vi "GTcode_v6 - WithEMGSubVI.vi"() -> ()   [LabVIEW 2016]
uses:
  <vilib>/Utility/config.llb/NI_LVConfig.lvlib
  <vilib>/Utility/config.llb/Write Key (U32).vi
  <vilib>/Utility/config.llb/Read Key (U32).vi
  <vilib>/Analysis/NI_AALBase.lvlib
  <vilib>/Utility/config.llb/Write Key (I32).vi
  <vilib>/Utility/config.llb/Write Key (String).vi
  <vilib>/Utility/config.llb/Read Key (I32).vi
  <vilib>/Utility/config.llb/Write Key (Double).vi
panel:
  in  "InitCH4 Path File":path=path "C:/Users/BUCKLEY-ADMIN/Desktop/DCScode_simulISS_MAP/flex05-4chPascal.dll"
  in  "Stop CH8":path=path "C:/Users/BUCKLEY-ADMIN/Desktop/DCScode_simulISS_MAP/flex05oem8chauto100nsPASCAL_win7.dll"
  in  "Stop Ch 4 Path":path=path "C:/Users/BUCKLEY-ADMIN/Desktop/DCScode_simulISS_MAP/flex05-4chPascal.dll"
  in  "FreeCh4 Path":path=path "C:/Users/BUCKLEY-ADMIN/Desktop/DCScode_simulISS_MAP/flex05-4chPascal.dll"
  in  "initCh4 path":path=path "C:/Users/BUCKLEY-ADMIN/Desktop/DCScode_simulISS_MAP/flex05-4chPascal.dll"
  in  "Ch8 Init channel":path=path "C:/Users/BUCKLEY-ADMIN/Desktop/DCScode_simulISS_MAP/flex05oem8chauto100nsPASCAL_win7.dll"
  in  "FreeCH8 Path":path=path "C:/Users/BUCKLEY-ADMIN/Desktop/DCScode_simulISS_MAP/flex05oem8chauto100nsPASCAL_win7.dll"
  in  "StartCH8 Path":path=path "C:/Users/BUCKLEY-ADMIN/Desktop/DCScode_simulISS_MAP/flex05oem8chauto100nsPASCAL_win7.dll"
  in  "StartCH4":path=path "C:/Users/BUCKLEY-ADMIN/Desktop/DCScode_simulISS_MAP/flex05-4chPascal.dll"
  in  "InitCh8 8 Dectectors Path":path=path "C:/Users/BUCKLEY-ADMIN/Desktop/DCScode_simulISS_MAP/flex05oem8chauto100nsPASCAL_win7.dll"
  in  "init CH4 path":path=path "C:/Users/BUCKLEY-ADMIN/Desktop/DCScode_simulISS_MAP/flex05-4chPascal.dll"
  in  "initCH8 Path":path
  in  "Tab Control":T1(tab)=enum."Real Time Fitting Parameters"
  out "Thermometer":dbl(slide) scale=0.0..100.0
  out "mean":dbl format="%0.1e"
  out "COV":dbl format="%0.1f"
  in  "Fixed Time":bool
  in  "Detector Used":T2(ring)=enum."Det 2"
  in  "Real Time Fitting?":bool=TRUE
  out "g2":cluster{"Delay Time":sgl[], sgl[]}[](graph) caption="Normalized Correlation Function"
  out "Tau":cluster{"tmp":dbl, dbl}(graph) caption="Relative Changes of Flow"
  in  "QUIT":bool
  in  "Clear plots":bool
  in  "Baseline":bool
  in  "MARK\nMark":bool
  in  "Stop":bool
  in  "Sequence Scan":bool
  out "Mark #":u32
  out "Trial #":u32
  out "Frame #":u32
  out "Det 8":sgl format="%.3f"
  out "Det 7":sgl format="%.3f"
  out "Det 6":sgl format="%.3f"
  out "Det 5":sgl format="%.3f"
  out "Det 4":sgl format="%.3f"
  out "Det 3":sgl format="%.3f"
  out "Det 2":sgl format="%.3f"
  out "Det 1":sgl format="%.3f"
  out "Computer Time":string="2010-1-12 23:16:10"
  in  "D1":bool
  in  "D2":bool
  in  "D3":bool
  in  "D4":bool
  in  "D5":bool
  in  "D6":bool
  in  "D7":bool
  in  "D8":bool
  out "Tau 2":T3(graph)={1.6593152555505744e-08, 3.9427894777554196e-08, 4.065716407938411e-08, 1.5135790977358522e-08, 2.4870420100428357e-08, 7.094765128107397e-08, 0.0, 4.1348620928852906e-07, 1.5886917674344795e-08, 4.0280526032721455e-08, -1.0, -1.0} caption="Blood Flow Index (cm2/s)"
  in  "Fixed # of Frames":u32=5
  out "Status":string="Quit"
  in  "Optical Switch OPEN":bool
  in  "Delay between frames(ms)":u32=500
  out "Time Left (ms)":sgl format="%.3f"
  in  "Integration Time (ms)":sgl=1000.0 min=1 max=13000 step=1
  in  "File\nName:":string="test0"
  in  "Data Save Directory:":path=path "C:/data"
  in  "ISS Lasers ON":bool
  in  "Test":bool
  in  "Lines":tag="Dev1/port1/line0:1, Dev1/port1/line3:7"
  in  "Delaytime(ms)":u32=200
  in  "Initialize Correlator":bool
  in  "Detector Select":enum32{"4 Detectors", "8 Detectors"}(radio)=enum."8 Detectors"
  in  "Update Time (ms)\nDO NOT CHANGE!":u32=105 min=1 max=999 step=1
  in  "Laser Input Name":refnum<visa-resource-name>="COM7"
  out "Flow in each detector":dbl[](array[numeric])=[-1.0, -1.0, -1.0, -1.0, -1.0, -1.0, -1.0, -1.0, -1.0, -1.0, -1.0, -1.0]
  in  "Visible Averages":bool[](array[boolean])=[FALSE, FALSE, FALSE, FALSE]
  in  "Avg":bool[][](array[boolean])=[[FALSE, FALSE, FALSE, FALSE, FALSE, FALSE, FALSE, FALSE], [FALSE, FALSE, FALSE, FALSE, FALSE, FALSE, FALSE, FALSE], [FALSE, FALSE, FALSE, FALSE, FALSE, FALSE, FALSE, FALSE], [FALSE, FALSE, FALSE, FALSE, FALSE, FALSE, FALSE, FALSE]]
  in  "rho":dbl[](array[numeric])=[2.5, 2.5, 2.5, 2.5, 2.5, 2.5, 2.5, 2.5, -1.0, -1.0, -1.0, -1.0]
  in  "Other Settings":u32[](array[numeric])=[1, 120, 0, 1] caption="Flow in each detector"
  in  "Initial Guess":dbl[](array[numeric])=[1e-08, 0.5, 0.05, 10.0] caption="Flow in each detector"
  in  "TrialDataFileExtension":string
  in  "UI Data Path":path=path "C:/Users/Tinggroup/Desktop/VRMuscleActivationVisualizer/LabviewFiles/Jake DCScode_GT/BiofeedbackEMGPackage/BiofeedbackData.txt"
  out "4CH?":bool
  out "Detector#":u32=1
  out "Source#":u32=1
  # "kHz"
  # "kHz"
  # "Don't Change these Parameters unless you know clearly what you are doing"
  # "ISS Triggers Setup"
  # "Channel Parameters"
  # "Step1"
  # "Line"
  # "0"
  # "1"
  # "3"
  # "4"
  # "5"
  # "6"
  # "7"
  # "*The number of lines in the list must\nmatch the number of elements in\nthe array."
  # "Step2"
  # "Line"
  # "0"
  # "1"
  # "3"
  # "4"
  # "5"
  # "6"
  # "7"
  # "Step3"
  # "Line"
  # "0"
  # "1"
  # "3"
  # "4"
  # "5"
  # "6"
  # "7"
  # "Line    Signal\n\n0           ISS Trigger (0: OFF, 1: ON)\n1           Flow Laser 1 ON/OFF (0:OFF, 1:ON)\n2           ISS Data Acquisition (0: DONE, 1: NO)\n3           ISS Laser ON/OFF (0: ON, 1: OFF)\n4           Trigger for Marks  (0: OFF, 1: ON)\n5           Flow Laser 2 ON/OFF (0:OFF, 1:ON)\n6           Reserved\n7           Reserved"
  # "Wait ISS Data Acuisition DONE Signal"
  # "Step4"
  # "Step5"
  # "Line"
  # "0"
  # "1"
  # "3"
  # "4"
  # "5"
  # "6"
  # "7"
  # "Flow Lasers Setup"
  # "FROM FRONT PANEL"
  # "Line"
  # "0"
  # "1"
  # "3"
  # "4"
  # "5"
  # "6"
  # "7"
  # "Line"
  # "0"
  # "1"
  # "3"
  # "4"
  # "5"
  # "6"
  # "7"
  # "Det 1"
  # "Det 2"
  # "Det 3"
  # "Det 4"
  # "Det 5"
  # "Det 6"
  # "Det 7"
  # "Det 8"
  # "Avg 1"
  # "Avg 2"
  # "Avg 3"
  # "Avg 4"
  # "Db"
  # "Beta"
  # "Mua"
  # "MuS'"
  # "1"
  # "2"
  # "3"
  # "4"
  # "5"
  # "6"
  # "7"
  # "8"
  # "Avg 1"
  # "Starting Pt"
  # "End Pt"
  # "Approximate"
  # "Variables"
  # "Avg 2"
  # "Avg 3"
  # "Avg 4"
  # "Source Detector  Separations"
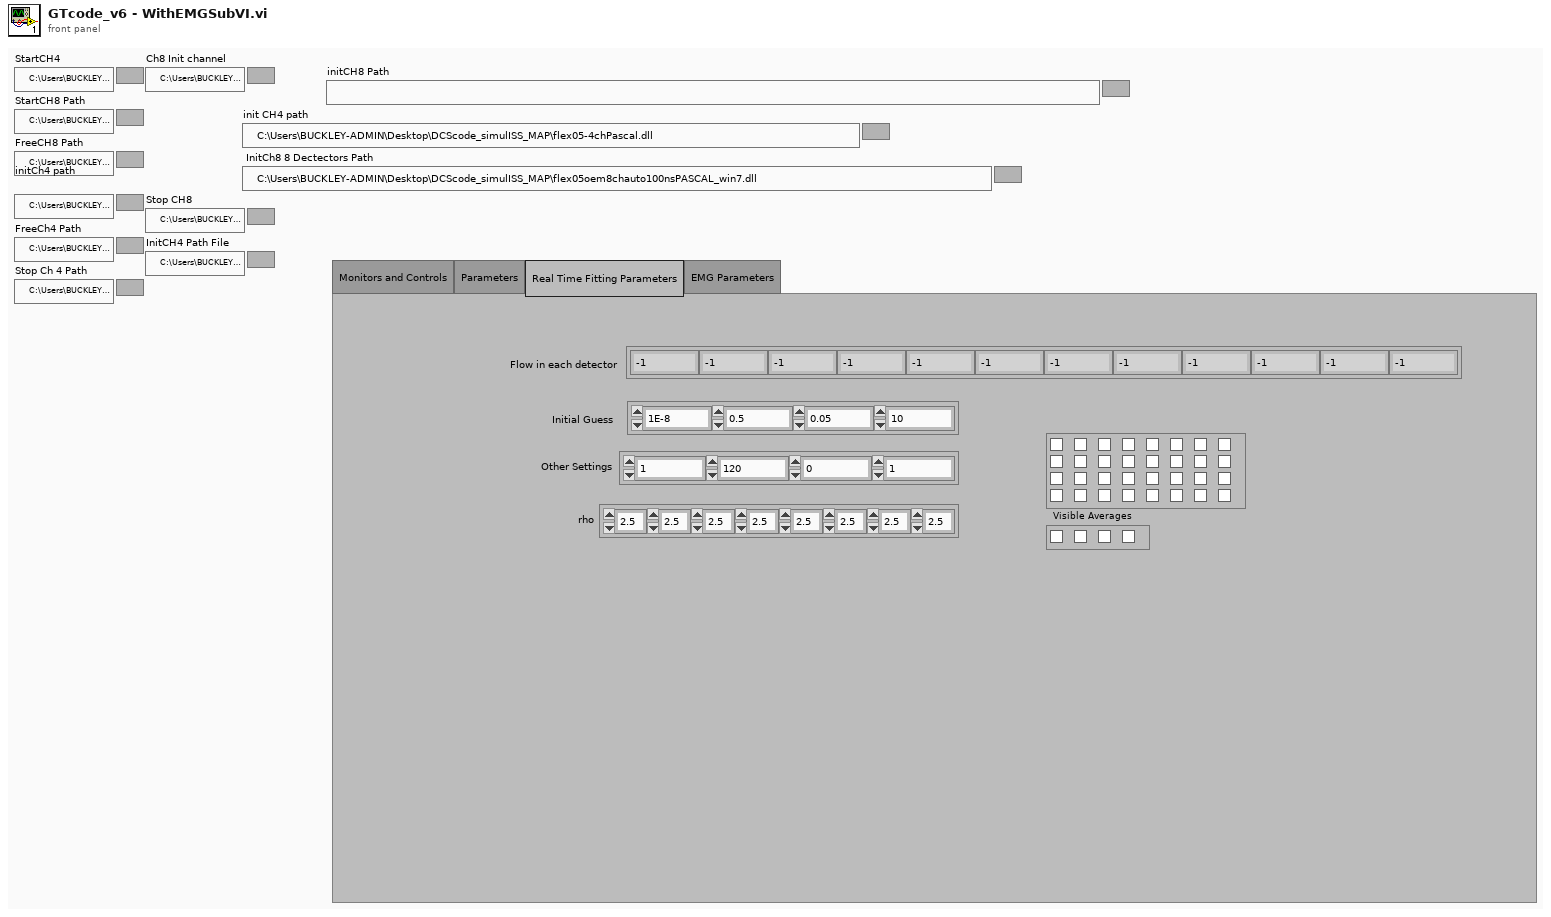
[diagram p1: front panel]
types:
  T1 = enum32{"Monitors and Controls", "Parameters", "Real Time Fitting Parameters", "EMG Parameters"}
  T2 = enum16{"Det 1", "Det 2", "Det 3", "Det 4", "Det 5", "Det 6", "Det 7", "Det 8"}
  T3 = cluster{dbl, dbl, dbl, dbl, dbl, dbl, dbl, dbl, dbl, dbl, dbl, dbl}
  T4 = enum8{"Enabled", "Disabled", "Disabled and Grayed Out"}
  T5 = cluster{dbl, dbl, dbl, dbl, dbl, dbl, dbl, dbl, dbl, dbl, dbl, dbl}[]
  T6 = typedef "NI_LVConfig.lvlib/Config Data RefNum.ctl" = refnum<k1>
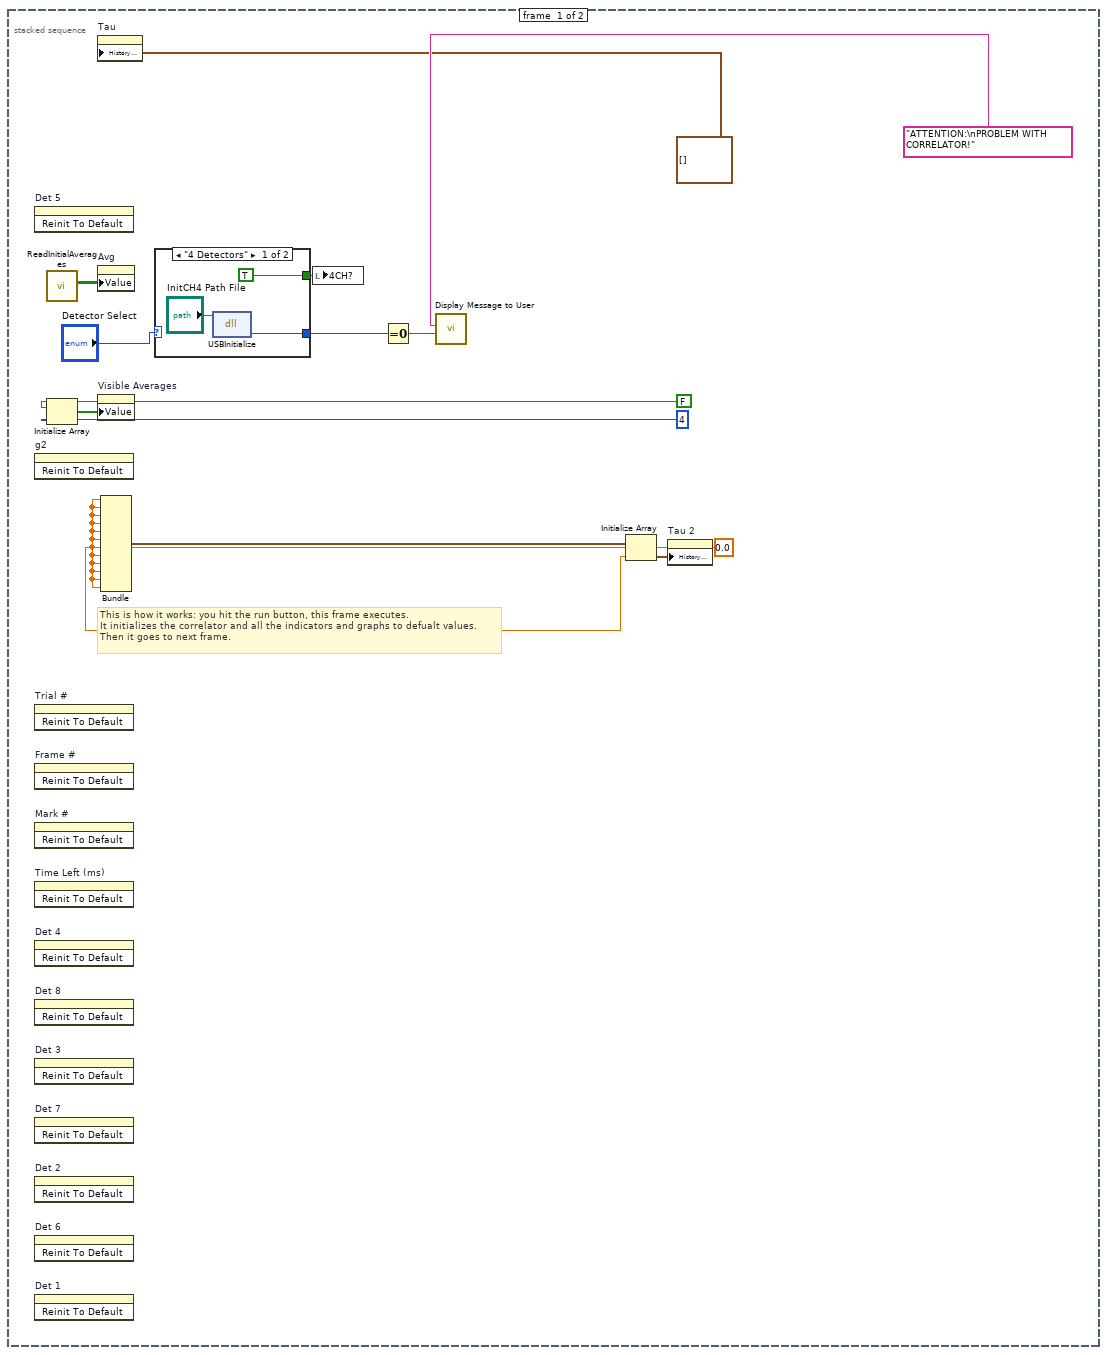
[diagram p2: hidden frame]
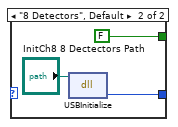
[diagram p3: hidden frame]
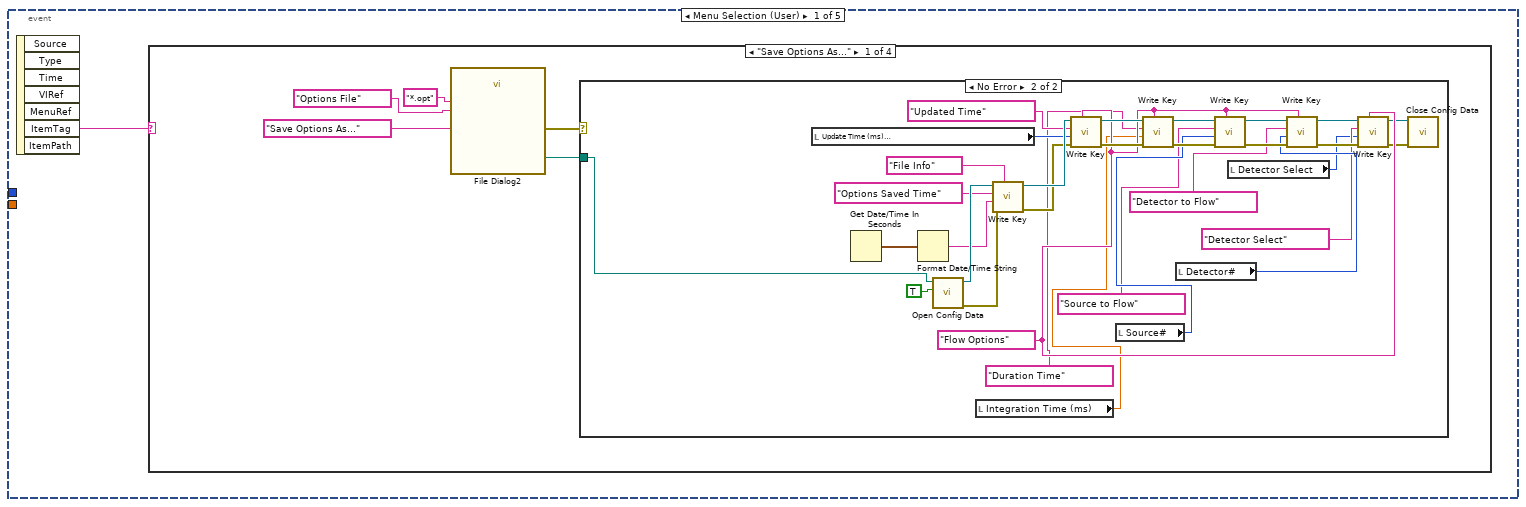
[diagram p5: hidden frame]
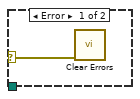
[diagram p6: hidden frame]
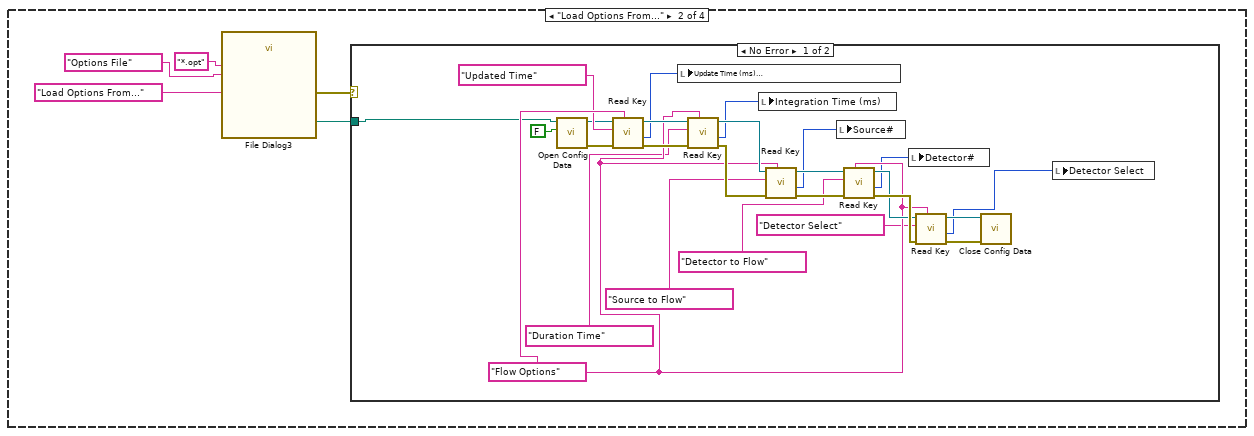
[diagram p7: hidden frame]
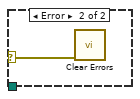
[diagram p8: hidden frame]
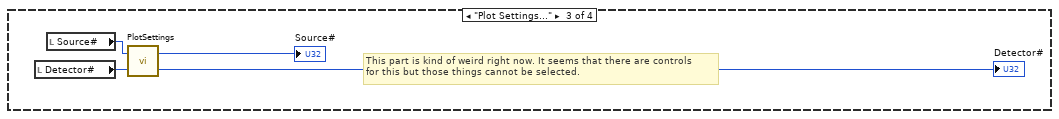
[diagram p9: hidden frame]
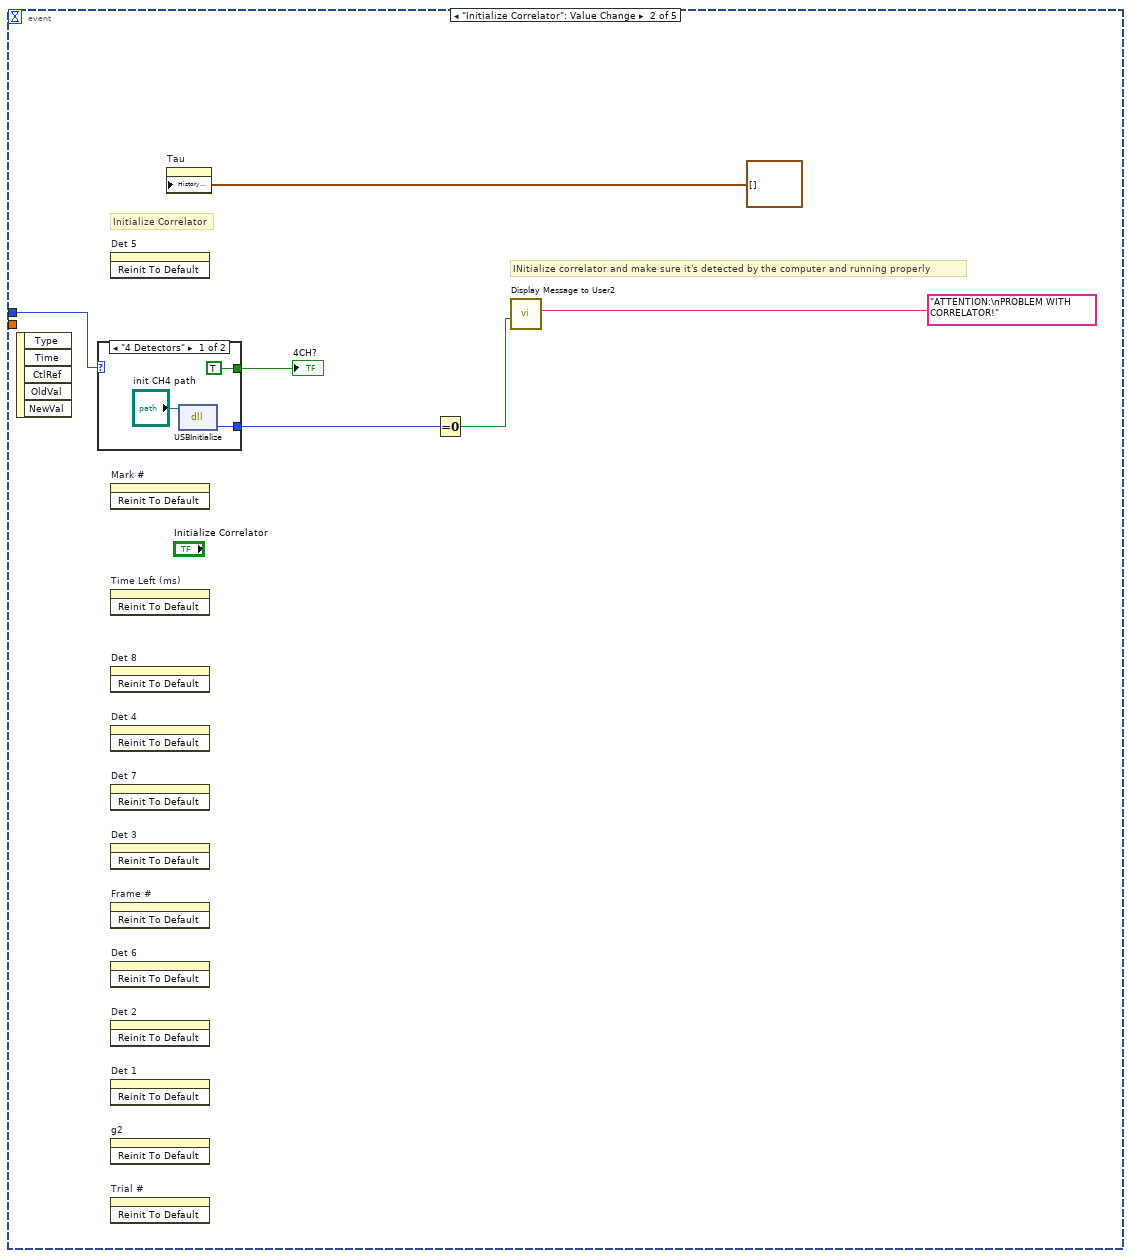
[diagram p11: hidden frame]
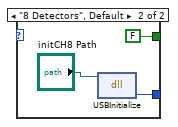
[diagram p12: hidden frame]
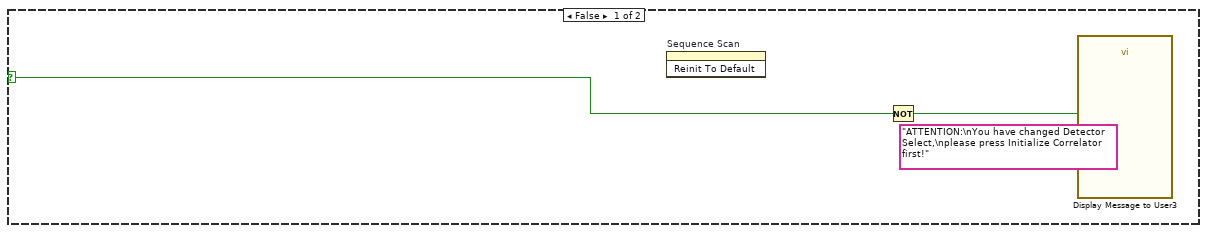
[diagram p13: hidden frame]
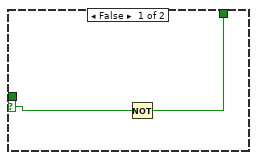
[diagram p14: hidden frame]
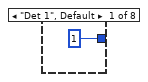
[diagram p20: hidden frame]
diagram:
  n1 = while {
    stop <- w7 stop-if-true
    n2 = local read "UI Data Path"() -> (w10:path)
    n3 = Read from Text File(file (use dialog)=w10) -> (text=w9:string)  [unwired: 3 in, 3 out]
    n4 = Fract/Exp String To Number(string=w9) -> (number=→"Thermometer":dbl)  [unwired: 3 in, 1 out]
    n5 = local read "Stop"() -> (w7:bool)
  }
  n6 = local read "Laser Input Name"() -> (w5:refnum<visa-resource-name>)
  n7 = local read "Data Save Directory:"() -> (w2:path)
  n8 = local read "File\nName:"() -> (w1:string)
  n9 = call "BioFeedback7(DAQ+8-channel)SubVIToUI.vi"("UI Data Input File"="UI Data Path", "Data Directory"=w2, "File Name"=w1, "Extension"="TrialDataFileExtension") -> ()  [unwired: 12 in]
  n10 = call "iBs.vi"("Laser On/Off"=FALSE, "VISA resource name"=w5) -> ()
  n11 = stacked-sequence {
    frame #0 {
      w13 = 0.0
      # "This is how it works: you hit the run button, this frame executes.\nIt initializes the correlator and all the indicators and graphs to defualt values.\nThen it goes to next frame."
      n12 = invoke on="Det 5" class="DigNum (strict)" method="Reinit To Default"() -> ()  [unwired: 3 in, 3 out]
      n13 = invoke on="g2" class="XYGraph (strict)" method="Reinit To Default"() -> ()  [unwired: 3 in, 3 out]
      n14 = invoke on="Trial #" class="DigNum (strict)" method="Reinit To Default"() -> ()  [unwired: 3 in, 3 out]
      n15 = invoke on="Frame #" class="DigNum (strict)" method="Reinit To Default"() -> ()  [unwired: 3 in, 3 out]
      n16 = invoke on="Mark #" class="DigNum (strict)" method="Reinit To Default"() -> ()  [unwired: 3 in, 3 out]
      n17 = invoke on="Time Left (ms)" class="DigNum (strict)" method="Reinit To Default"() -> ()  [unwired: 3 in, 3 out]
      n18 = invoke on="Det 4" class="DigNum (strict)" method="Reinit To Default"() -> ()  [unwired: 3 in, 3 out]
      n19 = invoke on="Det 8" class="DigNum (strict)" method="Reinit To Default"() -> ()  [unwired: 3 in, 3 out]
      n20 = invoke on="Det 3" class="DigNum (strict)" method="Reinit To Default"() -> ()  [unwired: 3 in, 3 out]
      n21 = invoke on="Det 7" class="DigNum (strict)" method="Reinit To Default"() -> ()  [unwired: 3 in, 3 out]
      n22 = invoke on="Det 2" class="DigNum (strict)" method="Reinit To Default"() -> ()  [unwired: 3 in, 3 out]
      n23 = invoke on="Det 6" class="DigNum (strict)" method="Reinit To Default"() -> ()  [unwired: 3 in, 3 out]
      n24 = invoke on="Det 1" class="DigNum (strict)" method="Reinit To Default"() -> ()  [unwired: 3 in, 3 out]
      n25 = call "ReadInitialAverages.vi"() -> ("avgOut"=w12:bool[][])  [unwired: 11 in]
      n26 = Initialize Array(FALSE, 4) -> (w11:bool[])
      n27 = property on="Tau" class="WFChart (strict)"("History Data"=cluster{"tmp":dbl, dbl}[] []) -> ()  [unwired: 2 in, 2 out]
      n28 = property on="Avg" class="Arr (strict)"("Value"=w12) -> ()  [unwired: 2 in, 2 out]
      n29 = property on="Visible Averages" class="Arr (strict)"("Value"=w11) -> ()  [unwired: 2 in, 2 out]
      n30 = Bundle(w13, w13, w13, w13, w13, w13, w13, w13, w13, w13, w13, w13) -> (w15:T3)  [unwired: 1 in]
      n31 = case shown="\"4 Detectors\"" "Detector Select" {
        tunnel: [w26 w29] -> w23
        tunnel: [TRUE FALSE] -> w21
        frame "4 Detectors" {
          n32 = dll-call lib="C:/Users/BUCKLEY-ADMIN/Desktop/DCScode_simulISS_MAP/flex05-4chPascal.dll" fn="USBInitialize" label="InitCH4"(path in="InitCH4 Path File") -> ("return type"=w26:u8)  [unwired: 2 in, 2 out]
        }
        frame "8 Detectors", Default {
          n33 = dll-call lib="C:/Users/BUCKLEY-ADMIN/Desktop/DCScode_simulISS_MAP/flex05oem8chauto100nsPASCAL_win7.dll" fn="USBInitialize" label="InitCH8"(path in="InitCh8 8 Dectectors Path") -> ("return type"=w29:u8)  [unwired: 2 in, 2 out]
        }
      }
      n34 = local write "4CH?"(w21) -> ()
      n35 = Equal To 0?(x=w23) -> (x = 0?=w22:bool)
      n36 = call "Display Message to User"("Enable"=w22, "Message"="ATTENTION:\nPROBLEM WITH CORRELATOR!") -> ()  [unwired: 8 in, 2 out]
      n37 = Initialize Array(w15, w13) -> (w14:T5)
      n38 = property on="Tau 2" class="WFChart (strict)"("History Data"=w14) -> ()  [unwired: 2 in, 2 out]
    }
    frame #1 {
      n39 = while {
        stop <- w33 stop-if-true
        # "Looks at whether using 4 or 8 ch correlator\nGenerates time points for g2 function based on correlator"
        n40 = local read "Detector Select"() -> (w31:enum32{"4 Detectors", "8 Detectors"})
        n41 = case shown="\"8 Detectors\"" w31 {
          tunnel: [_ w34] -> w30
          frame "4 Detectors", Default {
          }
          frame "8 Detectors" {
            n42 = formula code="int i,j;\nfloat DelayTime[256];\nfloat first_delay;\n\nfirst_delay = 2E-7;\n\nfor(i=0;i<16;i++)\nDelayTime[i] = (i+1)*first_delay;\nfor(j=1;j<31;j++)\n    for(i=0;i<8;i++)\n         DelayTime[i+(j-1)*8+16] = DelayTime[(j-1)*8+16+i-1]+first_delay*pow(2,j);"() -> ("DelayTime"=w34:dbl[])
          }
        }
        n43 = event shown="[2] \"Sequence Scan\": Value Change" {
          selector: _ -> [_ _ _ _ _]
          dyn-events: _ -> [_ _ _ _ _]
          timeout: 500 -> [_ _ _ _ _]
          tunnel: w30 -> [_ _ w126 _ _]
          tunnel: [_ _ _ "QUIT" _] -> w33
          tunnel: w31 -> [_ w111 w122 w614 _]
          event Menu Selection (User) {
            n44 = event-data() -> ("ItemTag"=w35:string)  [unwired: 1 in, 6 out]
            n45 = case shown="\"Save Options As...\"" w35 {
              frame "Save Options As..." {
                n46 = call "File Dialog2"("prompt"="Save Options As...", "pattern (all files)"="*.opt", "pattern label"="Options File") -> ("selected path"=w37:path, "error out"=w36:errorcluster)  [unwired: 9 in, 2 out]
                n47 = case shown="No Error" w36 {
                  selector: w36 -> [w41 _]
                  tunnel: w37 -> [_ w72]
                  frame Error {
                    n48 = call <vilib>:"Clear Errors.vi"("error in (no error)"=w41) -> ()  [unwired: 5 in, 2 out]
                  }
                  frame No Error {
                    w59 = "Flow Options"
                    n49 = local read "Update Time (ms)\nDO NOT CHANGE!"() -> (w52:u32)
                    n50 = Get Date/Time In Seconds() -> (seconds since 1Jan1904=w58:timestamp)
                    n51 = Format Date/Time String(seconds (now)=w58) -> (date/time string=w54:string)  [unwired: 2 in]
                    n52 = call <vilib>:"Open Config Data.vi"("create file if necessary (T)"=TRUE, "configuration file path"=w72) -> ("error out"=w70:errorcluster, "refnum"=w69:T6)  [unwired: 7 in, 1 out]
                    n53 = local read "Integration Time (ms)"() -> (w50:sgl)
                    n54 = call-poly <vilib>:"Write Key.vi"("section"="File Info", "error in (no error)"=w70, "value"=w54, "key"="Options Saved Time", "refnum"=w69) -> ("error out"=w56:errorcluster, "refnum out"=w57:T6)  [unwired: 4 in, 1 out]
                    n55 = call-poly <vilib>:"Write Key.vi"("section"=w59, "error in (no error)"=w56, "value"=w52, "key"="Updated Time", "refnum"=w57) -> ("error out"=w68:errorcluster, "refnum out"=w67:T6)  [unwired: 4 in, 1 out]
                    n56 = local read "Source#"() -> (w49:u32)
                    n57 = call-poly <vilib>:"Write Key.vi"("section"=w59, "error in (no error)"=w68, "value"=w50, "key"="Duration Time", "refnum"=w67) -> ("error out"=w63:errorcluster, "refnum out"=w64:T6)  [unwired: 4 in, 1 out]
                    n58 = local read "Detector#"() -> (w46:u32)
                    n59 = call-poly <vilib>:"Write Key.vi"("section"=w59, "error in (no error)"=w63, "value"=w49, "key"="Source to Flow", "refnum"=w64) -> ("error out"=w65:errorcluster, "refnum out"=w66:T6)  [unwired: 4 in, 1 out]
                    n60 = local read "Detector Select"() -> (w44:enum32{"4 Detectors", "8 Detectors"})
                    n61 = call-poly <vilib>:"Write Key.vi"("section"=w59, "error in (no error)"=w65, "value"=w46, "key"="Detector to Flow", "refnum"=w66) -> ("error out"=w62:errorcluster, "refnum out"=w61:T6)  [unwired: 4 in, 1 out]
                    n62 = call-poly <vilib>:"Write Key.vi"("section"=w59, "error in (no error)"=w62, "value"=w44, "key"="Detector Select", "refnum"=w61) -> ("error out"=w42:errorcluster, "refnum out"=w43:T6)  [unwired: 4 in, 1 out]
                    n63 = call <vilib>:"Close Config Data.vi"("error in (no error)"=w42, "refnum"=w43) -> ()  [unwired: 8 in, 2 out]
                  }
                }
              }
              frame "Load Options From..." {
                n64 = call "File Dialog3"("prompt"="Load Options From...", "pattern (all files)"="*.opt", "pattern label"="Options File") -> ("selected path"=w74:path, "error out"=w73:errorcluster)  [unwired: 9 in, 2 out]
                n65 = case shown="No Error" w73 {
                  selector: w73 -> [_ w103]
                  tunnel: w74 -> [w78 _]
                  frame No Error {
                    w93 = "Flow Options"
                    n66 = call <vilib>:"Open Config Data.vi"("create file if necessary (T)"=FALSE, "configuration file path"=w78) -> ("error out"=w85:errorcluster, "refnum"=w84:T6)  [unwired: 7 in, 1 out]
                    n67 = call-poly <vilib>:"Read Key.vi"("section"=w93, "error in (no error)"=w85, "key"="Updated Time", "refnum"=w84) -> ("error out"=w101:errorcluster, "value"=w83:u32, "refnum out"=w100:T6)  [unwired: 4 in, 1 out]
                    n68 = local write "Update Time (ms)\nDO NOT CHANGE!"(w83) -> ()
                    n69 = call-poly <vilib>:"Read Key.vi"("section"=w93, "error in (no error)"=w101, "key"="Duration Time", "refnum"=w100) -> ("error out"=w96:errorcluster, "value"=w82:i32, "refnum out"=w97:T6)  [unwired: 4 in, 1 out]
                    n70 = local write "Integration Time (ms)"(w82) -> ()
                    n71 = call-poly <vilib>:"Read Key.vi"("section"=w93, "error in (no error)"=w96, "key"="Source to Flow", "refnum"=w97) -> ("error out"=w98:errorcluster, "value"=w79:u32, "refnum out"=w99:T6)  [unwired: 4 in, 1 out]
                    n72 = local write "Source#"(w79) -> ()
                    n73 = call-poly <vilib>:"Read Key.vi"("section"=w93, "error in (no error)"=w98, "key"="Detector to Flow", "refnum"=w99) -> ("error out"=w95:errorcluster, "value"=w80:u32, "refnum out"=w94:T6)  [unwired: 4 in, 1 out]
                    n74 = local write "Detector#"(w80) -> ()
                    n75 = call-poly <vilib>:"Read Key.vi"("section"=w93, "error in (no error)"=w95, "key"="Detector Select", "refnum"=w94) -> ("error out"=w86:errorcluster, "value"=w81:u32, "refnum out"=w87:T6)  [unwired: 4 in, 1 out]
                    n76 = call <vilib>:"Close Config Data.vi"("error in (no error)"=w86, "refnum"=w87) -> ()  [unwired: 8 in, 2 out]
                    n77 = local write "Detector Select"(w81) -> ()
                  }
                  frame Error {
                    n78 = call <vilib>:"Clear Errors.vi"("error in (no error)"=w103) -> ()  [unwired: 5 in, 2 out]
                  }
                }
              }
              frame "Plot Settings..." {
                # "This part is kind of weird right now. It seems that there are controls\nfor this but those things cannot be selected."
                n79 = local read "Detector#"() -> (w105:u32)
                n80 = local read "Source#"() -> (w106:u32)
                n81 = call "PlotSettings.vi"("Detectorin"=w105, "Sourcein"=w106) -> ("Detector#"=→"Detector#":u32, "Source#"=→"Source#":u32)
              }
              frame Default {
              }
            }
          }
          event "Initialize Correlator": Value Change {
            # "INitialize correlator and make sure it's detected by the computer and running properly"
            # "Initialize Correlator"
            n82 = event-data() -> ()  [unwired: 1 in, 5 out]
            n83 = case shown="\"4 Detectors\"" w111 {
              tunnel: [w116 w119] -> w113
              tunnel: [TRUE FALSE] -> w110
              frame "4 Detectors" {
                n84 = dll-call lib="C:/Users/BUCKLEY-ADMIN/Desktop/DCScode_simulISS_MAP/flex05-4chPascal.dll" fn="USBInitialize" label="InitCH4"(path in="init CH4 path") -> ("return type"=w116:u8)  [unwired: 2 in, 2 out]
              }
              frame "8 Detectors", Default {
                n85 = dll-call lib="C:/Users/BUCKLEY-ADMIN/Desktop/DCScode_simulISS_MAP/flex05oem8chauto100nsPASCAL_win7.dll" fn="USBInitialize" label="InitCH8"(path in="initCH8 Path") -> ("return type"=w119:u8)  [unwired: 2 in, 2 out]
              }
            }
            "4CH?" <- w110
            n86 = invoke on="Det 5" class="DigNum (strict)" method="Reinit To Default"() -> ()  [unwired: 3 in, 3 out]
            n87 = invoke on="Mark #" class="DigNum (strict)" method="Reinit To Default"() -> ()  [unwired: 3 in, 3 out]
            n88 = invoke on="Time Left (ms)" class="DigNum (strict)" method="Reinit To Default"() -> ()  [unwired: 3 in, 3 out]
            n89 = invoke on="Det 8" class="DigNum (strict)" method="Reinit To Default"() -> ()  [unwired: 3 in, 3 out]
            n90 = invoke on="Det 4" class="DigNum (strict)" method="Reinit To Default"() -> ()  [unwired: 3 in, 3 out]
            n91 = invoke on="Det 7" class="DigNum (strict)" method="Reinit To Default"() -> ()  [unwired: 3 in, 3 out]
            n92 = invoke on="Det 3" class="DigNum (strict)" method="Reinit To Default"() -> ()  [unwired: 3 in, 3 out]
            n93 = invoke on="Frame #" class="DigNum (strict)" method="Reinit To Default"() -> ()  [unwired: 3 in, 3 out]
            n94 = invoke on="Det 6" class="DigNum (strict)" method="Reinit To Default"() -> ()  [unwired: 3 in, 3 out]
            n95 = invoke on="Det 2" class="DigNum (strict)" method="Reinit To Default"() -> ()  [unwired: 3 in, 3 out]
            n96 = invoke on="Det 1" class="DigNum (strict)" method="Reinit To Default"() -> ()  [unwired: 3 in, 3 out]
            n97 = invoke on="g2" class="XYGraph (strict)" method="Reinit To Default"() -> ()  [unwired: 3 in, 3 out]
            n98 = invoke on="Trial #" class="DigNum (strict)" method="Reinit To Default"() -> ()  [unwired: 3 in, 3 out]
            n99 = property on="Tau" class="WFChart (strict)"("History Data"=cluster{"tmp":dbl, dbl}[] []) -> ()  [unwired: 2 in, 2 out]
            n100 = Equal To 0?(x=w113) -> (x = 0?=w112:bool)
            n101 = call "Display Message to User2"("Enable"=w112, "Message"="ATTENTION:\nPROBLEM WITH CORRELATOR!") -> ()  [unwired: 8 in, 2 out]
          }
          event "Sequence Scan": Value Change {
            # "Initialize Baseline"
            n102 = event-data() -> ()  [unwired: 1 in, 6 out]
            n103 = case shown="\"8 Detectors\", Default" w122 {
              tunnel: [w609 w610] -> w121
              frame "4 Detectors" {
                n104 = local read "4CH?"() -> (w609:bool)
              }
              frame "8 Detectors", Default {
                # "Select whether using 4 or 8ch correlator"
                n105 = local read "4CH?"() -> (w611:bool)
                n106 = Not(x=w611) -> (.not. x?=w610:bool)
              }
            }
            n107 = case shown="True" w121 {
              selector: w121 -> [w128 _]
              tunnel: w126 -> [_ w142]
              tunnel: w122 -> [_ w143]
              tunnel: sgl 1.0 -> [_ w141]
              frame False {
                n108 = invoke on="Sequence Scan" class="Bool" method="Reinit To Default"() -> ()  [unwired: 3 in, 3 out]
                n109 = Not(x=w128) -> (.not. x?=w127:bool)
                n110 = call "Display Message to User3"("Enable"=w127, "Message"="ATTENTION:\nYou have changed Detector Select,\nplease press Initialize Correlator first!") -> ()  [unwired: 8 in, 2 out]
              }
              frame True {
                # "This part pauses and alerts user that test function is on. If test function is accepted then code runs but data is not saved (no timestamp either)."
                # "This checks for if the file already exists in the directory using the timing file. \n*If YES, then we don't do anything to the lasers. We just display message and wait for the user to input a new name and press sequence again.\n*If NO, then we proceed as per normal."
                n111 = local read "File\nName:"() -> (w137:string)
                n112 = case shown="True" "Test" {
                  selector: "Test" -> [w145 _]
                  tunnel: "Test" -> [_ w147]
                  tunnel: [w144 w146] -> w130
                  frame False {
                    n113 = Not(x=w145) -> (.not. x?=w144:bool)
                  }
                  frame True {
                    n114 = call "Test ON"("Enable"=w147) -> ("No - STOP"=w148:bool, "OK"=w146:bool)  [unwired: 15 in, 2 out]
                    n115 = local write "Stop"(w148) -> ()
                  }
                }
                n116 = local read "Data Save Directory:"() -> (w136:path)
                n117 = Concatenate Strings(w137, "_TIMING", ".dat") -> (w139:string)
                n118 = Build Path(base path=w136, name or relative path=w139) -> (appended path=w135:path)
                n119 = call <vilib>:"Check if File or Folder Exists.vi"("path"=w135) -> ("file or folder exists?"=w132:bool)  [unwired: 8 in, 2 out]
                n120 = Not(x=w132) -> (.not. x?=w134:bool)
                n121 = Not And(1:w130, 2:w134) -> (0:w133:bool)
                n122 = case shown="False" w133 {
                  tunnel: w143 -> [w162 _]
                  tunnel: w142 -> [w161 _]
                  tunnel: w141 -> [w160 _]
                  frame False {
                    # "Turn relay on so that Optical switch is open and LED indicator is ON"
                    # "When the START button is pressed, the ISS lasers turn off"
                    n123 = local read "Test"() -> (w149:bool)
                    n124 = case shown="False" w149 {
                      frame False {
                        # "This bit stores the time stamp."
                        n125 = local read "File\nName:"() -> (w163:string)
                        n126 = Get Date/Time In Seconds() -> (seconds since 1Jan1904=w165:timestamp)
                        n127 = local read "Data Save Directory:"() -> (w164:path)
                        n128 = Format Date/Time String(seconds (now)=w165) -> (date/time string=w171:string)  [unwired: 2 in]
                        n129 = Concatenate Strings(w163, "_TIMING", ".dat") -> (w168:string)
                        n130 = Build Path(base path=w164, name or relative path=w168) -> (appended path=w167:path)
                        n131 = Write to Text File(file (use dialog)=w167, text=w171) -> (refnum out=w170:refnum<file>, error out=w169:errorcluster)  [unwired: 2 in, 1 out]
                        n132 = Close File(refnum=w170, error in=w169) -> ()  [unwired: 2 out]
                      }
                      frame True {
                      }
                    }
                    n133 = Build Array(TRUE, TRUE) -> (w159:bool[])
                    n134 = Build Array(FALSE) -> (w156:bool[])
                    n135 = local read "Fixed # of Frames"() -> (w154:u32)
                    n136 = call "DAQ Assistant"("data"=w159) -> ()  [unwired: 17 in, 2 out]
                    n137 = call "DAQ Assistant7"("data"=w156) -> ()  [unwired: 17 in, 2 out]
                    n138 = Initialize Array "Initialize Array"(nan, w154) -> (w152:dbl[])
                    n139 = while {
                      tunnel: w162 -> [w206]
                      tunnel: w161 -> [w205]
                      tunnel: w160 -> [_]
                      shift-right: [w177] -> _
                      shift-left: w152 -> [w178]
                      stop <- w179 stop-if-true
                      # "Only runs Real Time Fitting if \nReal Time Fitting box is checked \nand test function is off."
                      # "After testing is complete, turn off the lasers and\nreset  the buttons."
                      n140 = for {
                        N: 1 -> [_]
                        tunnel: w205 -> [w247]
                        tunnel: w206 -> [w246]
                        tunnel: [w243] -> w179
                        tunnel: [w242] -> w203
                        tunnel: [w240] -> w183
                        tunnel: [w239] -> w182
                        tunnel: [w238] -> w181
                        # "The logic here may look funny but it works elegantly. No matter if you choose \"Use Both Lasers\", the AND output is always\nfalse the first time these two boxes run since Laser 1 Value is always false, and the default is to use flow laser 1.\nBUT, the trick is if you chose \"Use Both Laser\" This big for loop is gonna run twice, the second time it runs, \nthe laser 1 value is TRUE because it is set to TRUE by the second box when the big for loop ran the first time. Now, when\nthe output of AND is true, ISS laser no longer runs. Only flow laser two is turned on and we execute the for loop to the right."
                        # "These two boxes take care of the flow chart.\nIt turn on ISS laser first, then triggers it and turn it off.\nIf ISS data is ready, then we go on to flow lase."
                        # "This loop may seem useless but it acts as a block. \nThis block does all the data collection, plotting and writing the data\nto file"
                        n141 = case shown="\"8 Detectors\", Default" w246 {
                          selector: w246 -> [w606 w608]
                          tunnel: [w606 w608] -> w244
                          frame "4 Detectors" {
                            n142 = dll-call lib="C:/Users/BUCKLEY-ADMIN/Desktop/DCScode_simulISS_MAP/flex05-4chPascal.dll" fn="USBStart" label="StartCH4"(path in="StartCH4") -> ()  [unwired: 3 in, 2 out]
                          }
                          frame "8 Detectors", Default {
                            n143 = dll-call lib="C:/Users/BUCKLEY-ADMIN/Desktop/DCScode_simulISS_MAP/flex05oem8chauto100nsPASCAL_win7.dll" fn="USBStart" label="StartCH8"(path in="StartCH8 Path") -> ()  [unwired: 3 in, 2 out]
                          }
                        }
                        n144 = for {
                          N: 1 -> [_]
                          tunnel: w247 -> [w268]
                          tunnel: [w252] -> w243
                          tunnel: w244 -> [w257]
                          tunnel: [w260] -> w242
                          tunnel: "MARK\nMark" -> [w259]
                          tunnel: [w258] -> w240
                          tunnel: [w249] -> w239
                          tunnel: [w256] -> w238
                          w269 = FALSE
                          w278 = u8 2
                          # "Only saves data if\ntest function is off."
                          # "If Fixed # Frames check box is selected,\ncode will run for # of frames specified on \nfront panel and then call Stop button"
                          # "This for loop here acts as a block as well. It takes the relative \nflow data from UpdateData.vi and plot the data on the graph.\nWhen \"Baseline\" is selected,  the data point goes to 1. When\n\"Mark\" is selected, a point at positive infinity is plotted and a\nvertical line joining the point and the x axis if displayed."
                          n145 = while {
                            tunnel: [w459] -> w277
                            tunnel: [w429] -> w276
                            tunnel: [w430] -> w275
                            tunnel: [w433] -> w252
                            tunnel: [w460] -> w274
                            tunnel: w268 -> [w462]
                            tunnel: w257 -> [w435]
                            stop <- w464 stop-if-true
                            # "D4 Tail Alarm"
                            # "D2 Tail Alarm"
                            # "D8 Tail Alarm"
                            # "D7 Tail Alarm"
                            # "D6 Tail Alarm"
                            # "D5 Tail Alarm"
                            # "D3 Tail Alarm"
                            # "D1 Tail Alarm"
                            # "When press STOP, turn off DCS laser LED indicator is OFF"
                            n146 = Not(x="D4") -> (.not. x?=w448:bool)
                            n147 = Not(x="D8") -> (.not. x?=w444:bool)
                            n148 = Not(x="D5") -> (.not. x?=w447:bool)
                            n149 = Not(x="D1") -> (.not. x?=w451:bool)
                            n150 = Not(x="D6") -> (.not. x?=w446:bool)
                            n151 = Not(x="D2") -> (.not. x?=w436:bool)
                            n152 = Not(x="D7") -> (.not. x?=w445:bool)
                            n153 = Not(x="D3") -> (.not. x?=w449:bool)
                            n154 = case shown="True" "Stop" {
                              selector: "Stop" -> [w503 w509]
                              tunnel: [w503 w506] -> w433
                              frame False {
                              }
                              frame True {
                                n155 = call "Prompt User for Input"("Enable"=w509) -> ("Yes"=w506:bool)  [unwired: 17 in, 1 out]
                                n156 = Build Array(w506, FALSE) -> (w508:bool[])
                                n157 = call "DAQ Assistant2"("data"=w508) -> ()  [unwired: 17 in, 2 out]
                                n158 = local read "Laser Input Name"() -> (w504:refnum<visa-resource-name>)
                                n159 = call "iBs.vi"("Laser On/Off"=FALSE, "VISA resource name"=w504) -> ()
                              }
                            }
                            n160 = case shown="True" "Clear plots" {
                              frame False {
                              }
                              frame True {
                                n161 = invoke on="g2" class="XYGraph (strict)" method="Reinit To Default"() -> ()  [unwired: 3 in, 3 out]
                              }
                            }
                            n162 = case shown="False" w448 {
                              selector: w448 -> [w550 w555]
                              frame False {
                                n163 = property on="Tau 2" class="WFChart (strict)"("Active Plot"=u32 3) -> (error out=w552:errorcluster)  [unwired: 2 in, 1 out]
                                n164 = property on="g2" class="XYGraph (strict)"("Active Plot"=u32 3) -> (error out=w553:errorcluster)  [unwired: 2 in, 1 out]
                                n165 = property on="g2" class="XYGraph (strict)"(error in=w553, "Plot.Visible?"=w550) -> ()  [unwired: 1 in, 2 out]
                                n166 = property on="Tau 2" class="WFChart (strict)"(error in=w552, "Plot.Visible?"=w550) -> ()  [unwired: 1 in, 2 out]
                              }
                              frame True {
                                n167 = property on="Tau 2" class="WFChart (strict)"("Active Plot"=u32 3) -> (error out=w556:errorcluster)  [unwired: 2 in, 1 out]
                                n168 = property on="Tau 2" class="WFChart (strict)"(error in=w556, "Plot.Visible?"=w555) -> ()  [unwired: 1 in, 2 out]
                                n169 = property on="g2" class="XYGraph (strict)"("Active Plot"=u32 3) -> (error out=w558:errorcluster)  [unwired: 2 in, 1 out]
                                n170 = property on="g2" class="XYGraph (strict)"(error in=w558, "Plot.Visible?"=w555) -> ()  [unwired: 1 in, 2 out]
                              }
                            }
                            n171 = case shown="False" w444 {
                              selector: w444 -> [w510 w515]
                              frame False {
                                n172 = property on="Tau 2" class="WFChart (strict)"("Active Plot"=u32 7) -> (error out=w511:errorcluster)  [unwired: 2 in, 1 out]
                                n173 = property on="g2" class="XYGraph (strict)"("Active Plot"=u32 7) -> (error out=w513:errorcluster)  [unwired: 2 in, 1 out]
                                n174 = property on="g2" class="XYGraph (strict)"(error in=w513, "Plot.Visible?"=w510) -> ()  [unwired: 1 in, 2 out]
                                n175 = property on="Tau 2" class="WFChart (strict)"(error in=w511, "Plot.Visible?"=w510) -> ()  [unwired: 1 in, 2 out]
                              }
                              frame True {
                                n176 = property on="Tau 2" class="WFChart (strict)"("Active Plot"=u32 7) -> (error out=w517:errorcluster)  [unwired: 2 in, 1 out]
                                n177 = property on="Tau 2" class="WFChart (strict)"(error in=w517, "Plot.Visible?"=w515) -> ()  [unwired: 1 in, 2 out]
                                n178 = property on="g2" class="XYGraph (strict)"("Active Plot"=u32 7) -> (error out=w518:errorcluster)  [unwired: 2 in, 1 out]
                                n179 = property on="g2" class="XYGraph (strict)"(error in=w518, "Plot.Visible?"=w515) -> ()  [unwired: 1 in, 2 out]
                              }
                            }
                            n180 = case shown="False" w447 {
                              selector: w447 -> [w540 w545]
                              frame False {
                                n181 = property on="Tau 2" class="WFChart (strict)"("Active Plot"=u32 4) -> (error out=w542:errorcluster)  [unwired: 2 in, 1 out]
                                n182 = property on="g2" class="XYGraph (strict)"("Active Plot"=u32 4) -> (error out=w543:errorcluster)  [unwired: 2 in, 1 out]
                                n183 = property on="g2" class="XYGraph (strict)"(error in=w543, "Plot.Visible?"=w540) -> ()  [unwired: 1 in, 2 out]
                                n184 = property on="Tau 2" class="WFChart (strict)"(error in=w542, "Plot.Visible?"=w540) -> ()  [unwired: 1 in, 2 out]
                              }
                              frame True {
                                n185 = property on="Tau 2" class="WFChart (strict)"("Active Plot"=u32 4) -> (error out=w547:errorcluster)  [unwired: 2 in, 1 out]
                                n186 = property on="Tau 2" class="WFChart (strict)"(error in=w547, "Plot.Visible?"=w545) -> ()  [unwired: 1 in, 2 out]
                                n187 = property on="g2" class="XYGraph (strict)"("Active Plot"=u32 4) -> (error out=w548:errorcluster)  [unwired: 2 in, 1 out]
                                n188 = property on="g2" class="XYGraph (strict)"(error in=w548, "Plot.Visible?"=w545) -> ()  [unwired: 1 in, 2 out]
                              }
                            }
                            n189 = case shown="False" w451 {
                              selector: w451 -> [w580 w585]
                              frame False {
                                n190 = property on="Tau 2" class="WFChart (strict)"("Active Plot"=u32 0) -> (error out=w581:errorcluster)  [unwired: 2 in, 1 out]
                                n191 = property on="g2" class="XYGraph (strict)"("Active Plot"=u32 0) -> (error out=w583:errorcluster)  [unwired: 2 in, 1 out]
                                n192 = property on="g2" class="XYGraph (strict)"(error in=w583, "Plot.Visible?"=w580) -> ()  [unwired: 1 in, 2 out]
                                n193 = property on="Tau 2" class="WFChart (strict)"(error in=w581, "Plot.Visible?"=w580) -> ()  [unwired: 1 in, 2 out]
                              }
                              frame True {
                                n194 = property on="Tau 2" class="WFChart (strict)"("Active Plot"=u32 0) -> (error out=w587:errorcluster)  [unwired: 2 in, 1 out]
                                n195 = property on="Tau 2" class="WFChart (strict)"(error in=w587, "Plot.Visible?"=w585) -> ()  [unwired: 1 in, 2 out]
                                n196 = property on="g2" class="XYGraph (strict)"("Active Plot"=u32 0) -> (error out=w588:errorcluster)  [unwired: 2 in, 1 out]
                                n197 = property on="g2" class="XYGraph (strict)"(error in=w588, "Plot.Visible?"=w585) -> ()  [unwired: 1 in, 2 out]
                              }
                            }
                            n198 = case shown="False" w446 {
                              selector: w446 -> [w530 w535]
                              frame False {
                                n199 = property on="Tau 2" class="WFChart (strict)"("Active Plot"=u32 5) -> (error out=w532:errorcluster)  [unwired: 2 in, 1 out]
                                n200 = property on="g2" class="XYGraph (strict)"("Active Plot"=u32 5) -> (error out=w533:errorcluster)  [unwired: 2 in, 1 out]
                                n201 = property on="g2" class="XYGraph (strict)"(error in=w533, "Plot.Visible?"=w530) -> ()  [unwired: 1 in, 2 out]
                                n202 = property on="Tau 2" class="WFChart (strict)"(error in=w532, "Plot.Visible?"=w530) -> ()  [unwired: 1 in, 2 out]
                              }
                              frame True {
                                n203 = property on="Tau 2" class="WFChart (strict)"("Active Plot"=u32 5) -> (error out=w536:errorcluster)  [unwired: 2 in, 1 out]
                                n204 = property on="Tau 2" class="WFChart (strict)"(error in=w536, "Plot.Visible?"=w535) -> ()  [unwired: 1 in, 2 out]
                                n205 = property on="g2" class="XYGraph (strict)"("Active Plot"=u32 5) -> (error out=w538:errorcluster)  [unwired: 2 in, 1 out]
                                n206 = property on="g2" class="XYGraph (strict)"(error in=w538, "Plot.Visible?"=w535) -> ()  [unwired: 1 in, 2 out]
                              }
                            }
                            n207 = case shown="False" w436 {
                              selector: w436 -> [w570 w575]
                              frame False {
                                n208 = property on="Tau 2" class="WFChart (strict)"("Active Plot"=u32 1) -> (error out=w572:errorcluster)  [unwired: 2 in, 1 out]
                                n209 = property on="g2" class="XYGraph (strict)"("Active Plot"=u32 1) -> (error out=w573:errorcluster)  [unwired: 2 in, 1 out]
                                n210 = property on="g2" class="XYGraph (strict)"(error in=w573, "Plot.Visible?"=w570) -> ()  [unwired: 1 in, 2 out]
                                n211 = property on="Tau 2" class="WFChart (strict)"(error in=w572, "Plot.Visible?"=w570) -> ()  [unwired: 1 in, 2 out]
                              }
                              frame True {
                                n212 = property on="Tau 2" class="WFChart (strict)"("Active Plot"=u32 1) -> (error out=w577:errorcluster)  [unwired: 2 in, 1 out]
                                n213 = property on="Tau 2" class="WFChart (strict)"(error in=w577, "Plot.Visible?"=w575) -> ()  [unwired: 1 in, 2 out]
                                n214 = property on="g2" class="XYGraph (strict)"("Active Plot"=u32 1) -> (error out=w578:errorcluster)  [unwired: 2 in, 1 out]
                                n215 = property on="g2" class="XYGraph (strict)"(error in=w578, "Plot.Visible?"=w575) -> ()  [unwired: 1 in, 2 out]
                              }
                            }
                            n216 = case shown="False" w445 {
                              selector: w445 -> [w520 w525]
                              frame False {
                                n217 = property on="Tau 2" class="WFChart (strict)"("Active Plot"=u32 6) -> (error out=w522:errorcluster)  [unwired: 2 in, 1 out]
                                n218 = property on="g2" class="XYGraph (strict)"("Active Plot"=u32 6) -> (error out=w523:errorcluster)  [unwired: 2 in, 1 out]
                                n219 = property on="g2" class="XYGraph (strict)"(error in=w523, "Plot.Visible?"=w520) -> ()  [unwired: 1 in, 2 out]
                                n220 = property on="Tau 2" class="WFChart (strict)"(error in=w522, "Plot.Visible?"=w520) -> ()  [unwired: 1 in, 2 out]
                              }
                              frame True {
                                n221 = property on="Tau 2" class="WFChart (strict)"("Active Plot"=u32 6) -> (error out=w526:errorcluster)  [unwired: 2 in, 1 out]
                                n222 = property on="Tau 2" class="WFChart (strict)"(error in=w526, "Plot.Visible?"=w525) -> ()  [unwired: 1 in, 2 out]
                                n223 = property on="g2" class="XYGraph (strict)"("Active Plot"=u32 6) -> (error out=w528:errorcluster)  [unwired: 2 in, 1 out]
                                n224 = property on="g2" class="XYGraph (strict)"(error in=w528, "Plot.Visible?"=w525) -> ()  [unwired: 1 in, 2 out]
                              }
                            }
                            n225 = case shown="False" w449 {
                              selector: w449 -> [w560 w565]
                              frame False {
                                n226 = property on="Tau 2" class="WFChart (strict)"("Active Plot"=u32 2) -> (error out=w561:errorcluster)  [unwired: 2 in, 1 out]
                                n227 = property on="g2" class="XYGraph (strict)"("Active Plot"=u32 2) -> (error out=w563:errorcluster)  [unwired: 2 in, 1 out]
                                n228 = property on="g2" class="XYGraph (strict)"(error in=w563, "Plot.Visible?"=w560) -> ()  [unwired: 1 in, 2 out]
                                n229 = property on="Tau 2" class="WFChart (strict)"(error in=w561, "Plot.Visible?"=w560) -> ()  [unwired: 1 in, 2 out]
                              }
                              frame True {
                                n230 = property on="Tau 2" class="WFChart (strict)"("Active Plot"=u32 2) -> (error out=w567:errorcluster)  [unwired: 2 in, 1 out]
                                n231 = property on="Tau 2" class="WFChart (strict)"(error in=w567, "Plot.Visible?"=w565) -> ()  [unwired: 1 in, 2 out]
                                n232 = property on="g2" class="XYGraph (strict)"("Active Plot"=u32 2) -> (error out=w568:errorcluster)  [unwired: 2 in, 1 out]
                                n233 = property on="g2" class="XYGraph (strict)"(error in=w568, "Plot.Visible?"=w565) -> ()  [unwired: 1 in, 2 out]
                              }
                            }
                            n234 = Wait (ms)(milliseconds to wait="Update Time (ms)\nDO NOT CHANGE!") -> ()  [unwired: 1 out]
                            n235 = call "UpdateData.vi"("Duration Time (ms)"="Integration Time (ms)", "Detector Select"=w435, "Delay Time"=w462) -> ("Elapsed Time(s)"=w463:sgl, "Intensity Array"=w461:sgl[], "Tau Array"=w460:sgl[], "mean"=w425:dbl, "mean 8"=w405:dbl, "mean 2"=w374:dbl, "mean 7"=w406:dbl, "mean 3"=w410:dbl, "Intensity data"=w459:string, "g2 Display"=→"g2":cluster{"Delay Time":sgl[], sgl[]}[], "mean 4"=w409:dbl, "mean 5"=w408:dbl, "mean 6"=w407:dbl, "tau data"=w429:string, "g2 data"=w430:string)  [unwired: 2 in]
                            n236 = Multiply(x=sgl 1000.0, y=w463) -> (x*y=w467:sgl)
                            n237 = Less?(x=w425, y=1.005) -> (x < y?=w404:bool)
                            n238 = Less?(x=w374, y=1.005) -> (x < y?=w358:bool)
                            n239 = Less?(x=w410, y=1.005) -> (x < y?=w357:bool)
                            n240 = Less?(x=w409, y=1.005) -> (x < y?=w354:bool)
                            n241 = Less?(x=w408, y=1.005) -> (x < y?=w352:bool)
                            n242 = Less?(x=w407, y=1.005) -> (x < y?=w350:bool)
                            n243 = Less?(x=w406, y=1.005) -> (x < y?=w348:bool)
                            n244 = Less?(x=w405, y=1.005) -> (x < y?=w346:bool)
                            n245 = Index Array(array=w461, index #1=0, index #2=1, index #3=2, index #4=3, index #5=4, index #6=5, index #7=6, index #8=7) -> (element #1=w402:sgl, element #2=w381:sgl, element #3=w380:sgl, element #4=w379:sgl, element #5=w378:sgl, element #6=w377:sgl, element #7=w376:sgl, element #8=w375:sgl)
                            "Det 7" <- w376
                            "Det 6" <- w377
                            "Det 5" <- w378
                            "Det 4" <- w379
                            "Det 3" <- w380
                            "Det 2" <- w381
                            "Det 1" <- w402
                            "Det 8" <- w375
                            n246 = Subtract(x="Integration Time (ms)", y=w467) -> (x-y=w465:sgl)
                            "Time Left (ms)" <- w465
                            n247 = Greater?(x=w425, y=0.98) -> (0:w403:bool)
                            n248 = Greater?(x=w409, y=0.98) -> (0:w355:bool)
                            n249 = Greater?(x=w407, y=0.98) -> (0:w351:bool)
                            n250 = Greater?(x=w405, y=0.98) -> (0:w347:bool)
                            n251 = Greater Or Equal?(x=w402, y=sgl 2.0) -> (x >= y?=w399:bool)
                            n252 = Greater Or Equal?(x=w381, y=sgl 2.0) -> (x >= y?=w345:bool)
                            n253 = Greater Or Equal?(x=w380, y=sgl 2.0) -> (x >= y?=w343:bool)
                            n254 = Greater Or Equal?(x=w379, y=sgl 2.0) -> (x >= y?=w341:bool)
                            n255 = Greater Or Equal?(x=w378, y=sgl 2.0) -> (x >= y?=w339:bool)
                            n256 = Greater Or Equal?(x=w377, y=sgl 2.0) -> (x >= y?=w337:bool)
                            n257 = Less Or Equal?(x=w402, y=sgl 1000.0) -> (x <= y?=w398:bool)
                            n258 = Less Or Equal?(x=w381, y=sgl 1000.0) -> (x <= y?=w344:bool)
                            n259 = Less Or Equal?(x=w380, y=sgl 1000.0) -> (x <= y?=w342:bool)
                            n260 = Less Or Equal?(x=w379, y=sgl 1000.0) -> (x <= y?=w340:bool)
                            n261 = Less Or Equal?(x=w378, y=sgl 1000.0) -> (x <= y?=w338:bool)
                            n262 = Less Or Equal?(x=w377, y=sgl 1000.0) -> (x <= y?=w336:bool)
                            n263 = Less Or Equal?(x=w376, y=sgl 1000.0) -> (x <= y?=w334:bool)
                            n264 = Less Or Equal?(x=w375, y=sgl 1000.0) -> (x <= y?=w332:bool)
                            n265 = Greater Or Equal?(x=w376, y=sgl 2.0) -> (x >= y?=w335:bool)
                            n266 = Greater Or Equal?(x=w375, y=sgl 2.0) -> (x >= y?=w333:bool)
                            n267 = Greater?(x=w374, y=0.98) -> (0:w359:bool)
                            n268 = Greater?(x=w410, y=0.98) -> (0:w356:bool)
                            n269 = Greater?(x=w408, y=0.98) -> (0:w353:bool)
                            n270 = Greater?(x=w406, y=0.98) -> (0:w349:bool)
                            n271 = Build Array(w404, w403, w399, w398) -> (w397:bool[])
                            n272 = Build Array(w359, w358, w345, w344) -> (w373:bool[])
                            n273 = Build Array(w357, w356, w343, w342) -> (w372:bool[])
                            n274 = Build Array(w355, w354, w341, w340) -> (w371:bool[])
                            n275 = Build Array(w353, w352, w339, w338) -> (w370:bool[])
                            n276 = Build Array(w351, w350, w337, w336) -> (w369:bool[])
                            n277 = Build Array(w349, w348, w335, w334) -> (w368:bool[])
                            n278 = Build Array(w347, w346, w333, w332) -> (w367:bool[])
                            n279 = And Array Elements(Boolean array=w397) -> (logical AND=w396:bool)
                            n280 = And Array Elements(Boolean array=w373) -> (logical AND=w360:bool)
                            n281 = And Array Elements(Boolean array=w372) -> (logical AND=w361:bool)
                            n282 = And Array Elements(Boolean array=w371) -> (logical AND=w362:bool)
                            n283 = And Array Elements(Boolean array=w370) -> (logical AND=w363:bool)
                            n284 = And Array Elements(Boolean array=w369) -> (logical AND=w364:bool)
                            n285 = And Array Elements(Boolean array=w368) -> (logical AND=w365:bool)
                            n286 = And Array Elements(Boolean array=w367) -> (logical AND=w366:bool)
                            n287 = Less Or Equal To 0?(x=w465) -> (x <= 0?=w466:bool)
                            n288 = case shown="True" w396 {
                              frame False {
                                n289 = control-ref of="Det 1"() -> (w499:refnum<vi>)
                                n290 = property on="Property Node" class="Digital (strict)"(reference=w499, "DisabledEnum"=T4."Disabled and Grayed Out" ("Disabled")) -> ()  [unwired: 1 in, 2 out]
                              }
                              frame True {
                                n291 = control-ref of="Det 1"() -> (w501:refnum<vi>)
                                n292 = property on="Property Node" class="Digital (strict)"(reference=w501, "DisabledEnum"=T4."Enabled" ("Disabled")) -> ()  [unwired: 1 in, 2 out]
                              }
                            }
                            n293 = case shown="True" w360 {
                              frame False {
                                n294 = control-ref of="Det 2"() -> (w495:refnum<vi>)
                                n295 = property on="Property Node" class="Digital (strict)"(reference=w495, "DisabledEnum"=T4."Disabled and Grayed Out" ("Disabled")) -> ()  [unwired: 1 in, 2 out]
                              }
                              frame True {
                                n296 = control-ref of="Det 2"() -> (w497:refnum<vi>)
                                n297 = property on="Property Node" class="Digital (strict)"(reference=w497, "DisabledEnum"=T4."Enabled" ("Disabled")) -> ()  [unwired: 1 in, 2 out]
                              }
                            }
                            n298 = case shown="True" w361 {
                              frame False {
                                n299 = control-ref of="Det 3"() -> (w491:refnum<vi>)
                                n300 = property on="Property Node" class="Digital (strict)"(reference=w491, "DisabledEnum"=T4."Disabled and Grayed Out" ("Disabled")) -> ()  [unwired: 1 in, 2 out]
                              }
                              frame True {
                                n301 = control-ref of="Det 3"() -> (w493:refnum<vi>)
                                n302 = property on="Property Node" class="Digital (strict)"(reference=w493, "DisabledEnum"=T4."Enabled" ("Disabled")) -> ()  [unwired: 1 in, 2 out]
                              }
                            }
                            n303 = case shown="True" w362 {
                              frame False {
                                n304 = control-ref of="Det 4"() -> (w487:refnum<vi>)
                                n305 = property on="Property Node" class="Digital (strict)"(reference=w487, "DisabledEnum"=T4."Disabled and Grayed Out" ("Disabled")) -> ()  [unwired: 1 in, 2 out]
                              }
                              frame True {
                                n306 = control-ref of="Det 4"() -> (w489:refnum<vi>)
                                n307 = property on="Property Node" class="Digital (strict)"(reference=w489, "DisabledEnum"=T4."Enabled" ("Disabled")) -> ()  [unwired: 1 in, 2 out]
                              }
                            }
                            n308 = case shown="True" w363 {
                              frame False {
                                n309 = control-ref of="Det 5"() -> (w483:refnum<vi>)
                                n310 = property on="Property Node" class="Digital (strict)"(reference=w483, "DisabledEnum"=T4."Disabled and Grayed Out" ("Disabled")) -> ()  [unwired: 1 in, 2 out]
                              }
                              frame True {
                                n311 = control-ref of="Det 5"() -> (w485:refnum<vi>)
                                n312 = property on="Property Node" class="Digital (strict)"(reference=w485, "DisabledEnum"=T4."Enabled" ("Disabled")) -> ()  [unwired: 1 in, 2 out]
                              }
                            }
                            n313 = case shown="False" w364 {
                              frame False {
                                n314 = control-ref of="Det 6"() -> (w479:refnum<vi>)
                                n315 = property on="Property Node" class="Digital (strict)"(reference=w479, "DisabledEnum"=T4."Disabled and Grayed Out" ("Disabled")) -> ()  [unwired: 1 in, 2 out]
                              }
                              frame True {
                                n316 = control-ref of="Det 6"() -> (w481:refnum<vi>)
                                n317 = property on="Property Node" class="Digital (strict)"(reference=w481, "DisabledEnum"=T4."Enabled" ("Disabled")) -> ()  [unwired: 1 in, 2 out]
                              }
                            }
                            n318 = case shown="True" w365 {
                              frame False {
                                n319 = control-ref of="Det 7"() -> (w475:refnum<vi>)
                                n320 = property on="Property Node" class="Digital (strict)"(reference=w475, "DisabledEnum"=T4."Disabled and Grayed Out" ("Disabled")) -> ()  [unwired: 1 in, 2 out]
                              }
                              frame True {
                                n321 = control-ref of="Det 7"() -> (w477:refnum<vi>)
                                n322 = property on="Property Node" class="Digital (strict)"(reference=w477, "DisabledEnum"=T4."Enabled" ("Disabled")) -> ()  [unwired: 1 in, 2 out]
                              }
                            }
                            n323 = case shown="True" w366 {
                              frame False {
                                n324 = control-ref of="Det 8"() -> (w471:refnum<vi>)
                                n325 = property on="Property Node" class="Digital (strict)"(reference=w471, "DisabledEnum"=T4."Disabled and Grayed Out" ("Disabled")) -> ()  [unwired: 1 in, 2 out]
                              }
                              frame True {
                                n326 = control-ref of="Det 8"() -> (w473:refnum<vi>)
                                n327 = property on="Property Node" class="Digital (strict)"(reference=w473, "DisabledEnum"=T4."Enabled" ("Disabled")) -> ()  [unwired: 1 in, 2 out]
                              }
                            }
                            n328 = Or(x=w433, y=w466) -> (x .or. y?=w464:bool)
                            n329 = case shown="True" w464 {
                              tunnel: w435 -> [w590 _]
                              frame True {
                                n330 = case shown="\"8 Detectors\", Default" w590 {
                                frame "4 Detectors" {
                                n331 = dll-call lib="C:/Users/BUCKLEY-ADMIN/Desktop/DCScode_simulISS_MAP/flex05-4chPascal.dll" fn="USBStop" label="StopCH4"(path in="Stop Ch 4 Path") -> ()  [unwired: 3 in, 2 out]
                                }
                                frame "8 Detectors", Default {
                                n332 = dll-call lib="C:/Users/BUCKLEY-ADMIN/Desktop/DCScode_simulISS_MAP/flex05oem8chauto100nsPASCAL_win7.dll" fn="USBStop" label="StopCH8"(path in="Stop CH8") -> ()  [unwired: 3 in, 2 out]
                                }
                                }
                              }
                              frame False {
                              }
                            }
                          }
                          n333 = Current VI's Menubar() -> (w271:refnum<k9>)
                          n334 = local read "Trial #"() -> (w264:u32)
                          n335 = property on="QUIT" class="Bool"("Disabled"=w278) -> ()  [unwired: 2 in, 2 out]
                          n336 = Set Menu Item Info(7:"File", 9:w269, 11:w271) -> (3:w270:refnum<k9>)  [unwired: 4 in, 1 out]
                          n337 = Increment(x=w264) -> (x+1=w263:u32)
                          n338 = property on="Sequence Scan" class="Bool"("Disabled"=w278) -> ()  [unwired: 2 in, 2 out]
                          n339 = property on="Update Time (ms)\nDO NOT CHANGE!" class="DigNum (strict)"("Disabled"=w278) -> ()  [unwired: 2 in, 2 out]
                          n340 = property on="Integration Time (ms)" class="DigNum (strict)"("Disabled"=w278) -> ()  [unwired: 2 in, 2 out]
                          n341 = property on="Detector Select" class="RadioBtnsControl (strict)"("Disabled"=w278) -> ()  [unwired: 2 in, 2 out]
                          n342 = property on="Initialize Correlator" class="Bool"("Disabled"=w278) -> ()  [unwired: 2 in, 2 out]
                          n343 = local write "Trial #"(w263) -> ()
                          n344 = Set Menu Item Info(7:"Options", 9:w269, 11:w270) -> ()  [unwired: 4 in, 2 out]
                          n345 = case shown="\"Det 2\"" "Detector Used" {
                            tunnel: [1 2 3 4 5 6 7 8] -> w266
                            frame "Det 1", Default {
                            }
                            frame "Det 2" {
                            }
                            frame "Det 3" {
                            }
                            frame "Det 4" {
                            }
                            frame "Det 5" {
                            }
                            frame "Det 6" {
                            }
                            frame "Det 7" {
                            }
                            frame "Det 8" {
                            }
                          }
                          n346 = for {
                            N: 1 -> [_]
                            tunnel: w274 -> [w320]
                            tunnel: [w323] -> w267
                            tunnel: w266 -> [w322]
                            tunnel: w259 -> [w313]
                            n347 = case shown="True" w313 {
                              tunnel: [u32 0 w329] -> w323
                              frame False {
                              }
                              frame True {
                                n348 = local write "Trial #"(u32 0) -> ()
                                n349 = local read "Mark #"() -> (w331:u32)
                                n350 = Increment(x=w331) -> (x+1=w329:u32)
                                n351 = local write "Mark #"(w329) -> ()
                              }
                            }
                            n352 = Index Array(array=w320, index=w322) -> (element=w321:sgl)
                            n353 = Boolean To (0,1)(Boolean="Baseline") -> (0, 1=w325:i16)
                            n354 = case shown="False" w313 {
                              tunnel: [0.0 w327] -> w317
                              tunnel: inf -> [_ w327]
                              frame False {
                              }
                              frame True {
                              }
                            }
                            n355 = feedback #1() -> (w318:sgl)  [unwired: 1 in]
                            n356 = formula code="if(Tau==0) Tau=Tau+0.001;\nif(T==1) baselineflow=Tau;\n\ntmp=baselineflow/Tau;"("Tau"=w321, "T"=w325, "baselineflow"=w318) -> ("tmp"=w315:dbl, "baselineflow"=w319:sgl)
                            n357 = feedback-in #1(w319) -> ()
                            n358 = Bundle("tmp"=w315, w317) -> (→"Tau":cluster{"tmp":dbl, dbl})  [unwired: 1 in]
                          }
                          n359 = property on="Frame #" class="DigNum (strict)"() -> ("Value"=w250:u32)  [unwired: 2 in, 2 out]
                          n360 = case shown="True" "Fixed Time" {
                            tunnel: w250 -> [w301 w304]
                            tunnel: [w301 w304] -> w249
                            frame False {
                            }
                            frame True {
                              n361 = Less Or Equal?(x="Fixed # of Frames", y=w304) -> (x <= y?=w302:bool)
                              n362 = local write "Stop"(w302) -> ()
                            }
                          }
                          n363 = case shown="\"8 Detectors\", Default" w257 {
                            tunnel: w267 -> [w600 w604]
                            tunnel: [w601 w603] -> w284
                            tunnel: [4 8] -> w256
                            frame "4 Detectors" {
                              n364 = Build Array(w600, w600, w600, w600, w600) -> (w601:u32[])
                            }
                            frame "8 Detectors", Default {
                              n365 = Build Array(w604, w604, w604, w604, w604, w604, w604, w604, w604) -> (w603:u32[])
                            }
                          }
                          n366 = case shown="\"8 Detectors\", Default" w257 {
                            tunnel: ["%Duration\tID1\t\tID2\t\tID3\t\tID4\n" "%Duration\tID1\t\tID2\t\tID3\t\tID4\t\tID5\t\tID6\t\tID7\t\tID8\n"] -> w281
                            tunnel: ["%Tau\t\tTau1\t\tTau2\t\tTau3\t\tTau4\n" "%Tau\t\tTau1\t\tTau2\t\tTau3\t\tTau4\t\tTau5\t\tTau6\t\tTau7\t\tTau8\n"] -> w280
                            tunnel: ["%Delaytime\tD1\t\tD2\t\tD3\t\tD4\n" "%Delaytime\tD1\t\tD2\t\tD3\t\tD4\t\tD5\t\tD6\t\tD7\t\tD8\n"] -> w279
                            frame "4 Detectors" {
                            }
                            frame "8 Detectors", Default {
                            }
                          }
                          n367 = Increment(x=w249) -> (x+1=w251:u32)
                          n368 = Number To Decimal String(number=w249) -> (decimal integer string=w285:string)  [unwired: 1 in]
                          n369 = local write "Frame #"(w251) -> ()
                          n370 = Get Date/Time In Seconds() -> (seconds since 1Jan1904=w294:timestamp)
                          n371 = Array To Spreadsheet String(array=w284, 3:"%d") -> (spreadsheet string=w282:string)  [unwired: 1 in]
                          n372 = Format Date/Time String(seconds (now)=w294) -> (date/time string=w291:string)  [unwired: 2 in]
                          "Computer Time" <- w291
                          n373 = Concatenate Strings("File\nName:", "_flow_", w285, ".dat") -> (w254:string)
                          n374 = local read "Test"() -> (w248:bool)
                          n375 = Concatenate Strings("%", w291, "\r\n", w281, w277, w280, "%\t\t", w276, w279, w275, w282) -> (w262:string)
                          n376 = Build Path(base path="Data Save Directory:", name or relative path=w254) -> (appended path=w261:path)
                          n377 = case shown="False" w248 {
                            tunnel: w262 -> [w298 _]
                            tunnel: w261 -> [w297 _]
                            tunnel: [w296 _] -> w260
                            tunnel: [w295 _] -> w258
                            frame False {
                              n378 = Write to Text File(file (use dialog)=w297, text=w298) -> (refnum out=w299:refnum<file>, error out=w300:errorcluster)  [unwired: 2 in, 1 out]
                              n379 = Close File(refnum=w299, error in=w300) -> (path=w296:path, error out=w295:errorcluster)
                            }
                            frame True {
                            }
                          }
                        }
                      }
                      n380 = Index Array(array="Visible Averages", index=3) -> (element=w197:bool)
                      n381 = Index Array(array="Visible Averages", index=1) -> (element=w198:bool)
                      n382 = Index Array(array="Visible Averages", index=0) -> (element=w191:bool)
                      n383 = Index Array(array="Visible Averages", index=2) -> (element=w192:bool)
                      n384 = property on="Tau 2" class="WFChart (strict)"("Active Plot"=u32 11) -> (error out=w195:errorcluster)  [unwired: 2 in, 1 out]
                      n385 = property on="Tau 2" class="WFChart (strict)"("Active Plot"=u32 9) -> (error out=w200:errorcluster)  [unwired: 2 in, 1 out]
                      n386 = property on="Tau 2" class="WFChart (strict)"("Active Plot"=u32 8) -> (error out=w189:errorcluster)  [unwired: 2 in, 1 out]
                      n387 = property on="Tau 2" class="WFChart (strict)"("Active Plot"=u32 10) -> (error out=w194:errorcluster)  [unwired: 2 in, 1 out]
                      n388 = property on="Tau 2" class="WFChart (strict)"(error in=w195, "Plot.Visible?"=w197) -> ()  [unwired: 1 in, 2 out]
                      n389 = property on="Tau 2" class="WFChart (strict)"(error in=w200, "Plot.Visible?"=w198) -> ()  [unwired: 1 in, 2 out]
                      n390 = property on="Tau 2" class="WFChart (strict)"(error in=w189, "Plot.Visible?"=w191) -> ()  [unwired: 1 in, 2 out]
                      n391 = property on="Tau 2" class="WFChart (strict)"(error in=w194, "Plot.Visible?"=w192) -> ()  [unwired: 1 in, 2 out]
                      n392 = local read "Test"() -> (w175:bool)
                      n393 = Not(x=w175) -> (.not. x?=w174:bool)
                      n394 = Unbundle By Name(w183) -> ("status"=w202:bool)
                      n395 = for {
                        N: 1 -> [_]
                        tunnel: w203 -> [_]
                        n396 = local write "Stop"(FALSE) -> ()
                        n397 = Wait (ms)(milliseconds to wait="Delay between frames(ms)") -> ()  [unwired: 1 out]
                      }
                      n398 = And(x="Real Time Fitting?", y=w174) -> (x .and. y?=w173:bool)
                      n399 = Not(x=w202) -> (.not. x?=w201:bool)
                      n400 = case shown="True" w173 {
                        tunnel: w201 -> [_ w212]
                        tunnel: w182 -> [_ w211]
                        tunnel: w181 -> [_ w210]
                        tunnel: w178 -> [w207 w209]
                        tunnel: [w207 w208] -> w177
                        frame False {
                        }
                        frame True {
                          n401 = case shown="True" w212 {
                            tunnel: w211 -> [_ w232]
                            tunnel: w210 -> [_ w228]
                            tunnel: w209 -> [w213 w224]
                            tunnel: [w213 w222] -> w208
                            frame False {
                            }
                            frame True {
                              # "Initialize Array of NaNs with size of \"fixed number of frames, \nand run this array into the case structure by putting it \nthrough a shift register with each loop it will replace one of \nthe NaNs by the flow data of the detector used. Then this data\nis averaged and COV is calculated."
                              n402 = property on="Data Save Directory:" class="Path"() -> ("Value"=w234:path)  [unwired: 2 in, 2 out]
                              n403 = property on="File\nName:" class="Str"() -> ("Value"=w235:string)  [unwired: 2 in, 2 out]
                              n404 = call "GetFilePath.vi"("path"=w234, "file name"=w235, "frame number"=w232) -> ("final path C"=w227:string)  [unwired: 10 in, 2 out]
                              n405 = property on="Avg" class="Arr (strict)"() -> ("Value"=w233:bool[][])  [unwired: 2 in, 2 out]
                              n406 = call "DCSAnalysis.vi"("# Detectors"=w228, "File path"=w227, "Frame #"=w232, "rho"="rho", "other settings"="Other Settings", "avgBool"=w233, "var values"="Initial Guess") -> ("Flow in each detector"=w225:dbl[], "Tau"=→"Tau 2":T3)  [unwired: 17 in, 2 out]
                              "Flow in each detector" <- w225
                              n407 = local read "Detector Used"() -> (w214:T2)
                              n408 = local read "Trial #"() -> (w220:u32)
                              n409 = Decrement(x=w220) -> (x-1=w221:u32)
                              n410 = Index Array(array=w225, index=w214) -> (element=w223:dbl)
                              n411 = Replace Array Subset(array=w224, new element=w223, index=w221) -> (w222:dbl[])
                              n412 = call <vilib>:"Std Deviation and Variance.vi"("X"=w222) -> ("mean"=w218:dbl, "standard deviation"=w219:dbl)  [unwired: 1 in, 1 out]
                              "mean" <- w218
                              n413 = Divide(x=w219, y=w218) -> (x/y=w216:dbl)
                              n414 = Multiply(x=w216, y=100.0) -> (x*y=→"COV":dbl)
                            }
                          }
                        }
                      }
                    }
                    n415 = call "iBs.vi"("Laser On/Off"=TRUE, "VISA resource name"="Laser Input Name") -> ()
                  }
                  frame True {
                    n416 = invoke on="Sequence Scan" class="Bool" method="Reinit To Default"() -> ()  [unwired: 3 in, 3 out]
                    n417 = call "Display Message to User5"() -> ()  [unwired: 10 in, 2 out]
                  }
                }
              }
            }
            "Frame #" <- u32 0
            "Mark #" <- u32 0
            "Trial #" <- u32 0
          }
          event "QUIT": Value Change {
            # "Reset correlator before quitting"
            n418 = event-data() -> ()  [unwired: 1 in, 6 out]
            n419 = case shown="\"4 Detectors\"" w614 {
              frame "4 Detectors" {
                n420 = dll-call lib="C:/Users/BUCKLEY-ADMIN/Desktop/DCScode_simulISS_MAP/flex05-4chPascal.dll" fn="USBInitialize" label="InitCH4"(path in="initCh4 path") -> (error out=w618:errorcluster)  [unwired: 3 in, 1 out]
                n421 = dll-call lib="C:/Users/BUCKLEY-ADMIN/Desktop/DCScode_simulISS_MAP/flex05-4chPascal.dll" fn="USBFree" label="FreeCH4"(path in="FreeCh4 Path", error in=w618) -> ()  [unwired: 2 in, 2 out]
              }
              frame "8 Detectors", Default {
                n422 = dll-call lib="C:/Users/BUCKLEY-ADMIN/Desktop/DCScode_simulISS_MAP/flex05oem8chauto100nsPASCAL_win7.dll" fn="USBInitialize" label="InitCH8"(path in="Ch8 Init channel") -> (error out=w621:errorcluster)  [unwired: 3 in, 1 out]
                n423 = dll-call lib="C:/Users/BUCKLEY-ADMIN/Desktop/DCScode_simulISS_MAP/flex05oem8chauto100nsPASCAL_win7.dll" fn="USBFree" label="FreeCH8"(path in="FreeCH8 Path", error in=w621) -> ()  [unwired: 2 in, 2 out]
              }
            }
            n424 = local write "Status"("Quit") -> ()
            n425 = local write "Status"("Quit") -> ()
          }
          event Timeout {
            w626 = TRUE
            w625 = u8 0
            # "This case structure turns on\n      and off the ISS Lasers"
            # "This case structure ensures that when the\noptical switch is turned on, the relay tells \nthe laser to power on."
            # "The system sits here and wait for some buttons to be pressed. And the status is always \"waiting\". Once some button is pressed, this value driven event\nstructure goes to the appropriate frame."
            n426 = event-data() -> ()  [unwired: 1 in, 3 out]
            n427 = local write "Status"("Waiting") -> ()
            n428 = property on="MARK\nMark" class="Bool"("DisabledEnum"=w625) -> ()  [unwired: 2 in, 2 out]
            n429 = property on="QUIT" class="Bool"("Disabled"=w625) -> ()  [unwired: 2 in, 2 out]
            n430 = property on="Sequence Scan" class="Bool"("Disabled"=w625) -> ()  [unwired: 2 in, 2 out]
            n431 = property on="Initialize Correlator" class="Bool"("Disabled"=w625) -> ()  [unwired: 2 in, 2 out]
            n432 = property on="Update Time (ms)\nDO NOT CHANGE!" class="DigNum (strict)"("Disabled"=w625) -> ()  [unwired: 2 in, 2 out]
            n433 = property on="Integration Time (ms)" class="DigNum (strict)"("Disabled"=w625) -> ()  [unwired: 2 in, 2 out]
            n434 = property on="Detector Select" class="RadioBtnsControl (strict)"("Disabled"=w625) -> ()  [unwired: 2 in, 2 out]
            n435 = case shown="True" "ISS Lasers ON" {
              frame False {
                n436 = Build Array(FALSE) -> (w633:bool[])
                n437 = call "DAQ Assistant5"("data"=w633) -> ()  [unwired: 17 in, 2 out]
              }
              frame True {
                # "For Toptica laser control"
                n438 = local read "Laser Input Name"() -> (w635:refnum<visa-resource-name>)
                n439 = call "iBs.vi"("Laser On/Off"=TRUE, "VISA resource name"=w635) -> ()
                n440 = Build Array(TRUE) -> (w637:bool[])
                n441 = call "DAQ Assistant6"("data"=w637) -> ()  [unwired: 17 in, 2 out]
              }
            }
            n442 = case shown="True" "Optical Switch OPEN" {
              frame False {
                # "Send 2 signals, one for LED indicator, one for switch"
                n443 = Build Array(FALSE, FALSE) -> (w639:bool[])
                n444 = call "DAQ Assistant3"("data"=w639) -> ()  [unwired: 17 in, 2 out]
              }
              frame True {
                n445 = Build Array(TRUE, TRUE) -> (w642:bool[])
                n446 = call "DAQ Assistant4"("data"=w642) -> ()  [unwired: 17 in, 2 out]
              }
            }
            n447 = Current VI's Menubar() -> (w628:refnum<k9>)
            n448 = Set Menu Item Info(7:"File", 9:w626, 11:w628) -> (3:w627:refnum<k9>)  [unwired: 4 in, 1 out]
            n449 = Get Date/Time In Seconds() -> (seconds since 1Jan1904=w631:timestamp)
            n450 = Set Menu Item Info(7:"Options", 9:w626, 11:w627) -> ()  [unwired: 4 in, 2 out]
            n451 = Format Date/Time String(seconds (now)=w631) -> (date/time string=w632:string)  [unwired: 2 in]
            n452 = local write "Computer Time"(w632) -> ()
          }
        }
      }
    }
  }
